vi "SendCmd.vi"(0 "Axis In":T2, 1 "Data Length Constant (0)":u8, 5 "Command":T5 items=["Home Position"=201, "Preset Position"=13, "Soft Overtravel Enable/Disable"=221, "Drive Status"=115, "Position Command"=128, "Run Status"=117, "Fault Status"=116, "Position Error"=129, "Auto-Start Homing"=196, "Start Homing"=205, "Homing Type"=197, "Monitor Index Count"=173, "Motor Position"=126, "Velocity Motor"=133, "Power-Up Status"=1, "Drive Name"=6, "Position Window Size"=22, "Position Window Time"=23, "Zero Speed Limit"=34, "Speed Window Size"=35, "Up to Speed Limit"=37, "Forward Current Limit"=47, "Reverse Current Limit"=48, "Override Mode"=67, "Operation Mode"=90, "Host Control Mode"=97, "Reset Drive"=106, "Drive Enable"=107, "Setpoint Current"=108, "Setpoint Velocity"=109, "Setpoint Acceleration"=110, "Reset Faults"=111, "Position Comparator"=349, "Postition Comparator Polarity"=350, "Position Rollover Enable"=404, "Baud Rate"=80, "Frame Format"=81, "Drive Address"=82, "Broadcast Address"=83, "Auto-start Indexing"=88, "Start Index"=112, "Host Index"=184, "Index Type"=174, "Index Dist/Pos"=175, "Index Reg Dist"=176, "Index Velocity"=177, "Index Acceleration"=178, "Index Deceleration"=179, "Index Dwell"=180, "Index Count"=181, "Index Termination"=182, "Index Pointer"=183, "Index Abort Deceleration"=185, "Positive Soft Pos Limit"=216, "Define Home"=113, "Negative Soft Pos Limit"=217], 7 "Function":T4 items=["Read Working Value", "Write Working Value", "Read Non-Volatile Value", "Write Non-Volatile and Woring Value", "Copy Non-Volatile Value to Working Value", "Copy Working Value to Non-Volatile Value", "Read Default Value", "Copy Default Value to Non-Volatile and Working Values", "Read Min Value", "Read Max Value", "Read Array Index Min", "Read Array Index Max"], 9 "Data (0)":i32, 11 "error in (no error)":errorcluster, 12 "Index (0)":T3) -> (4 "Axis Out":T2, 6 "Data":i32, 10 "Error Message":T1 items=["Invalid Data"=1, "Command Not Enabled"=2, "EEPROM Write Error"=3, "Data Below Min"=4, "Data Above Max"=5, "Command Disabled when Drive Enabled"=6, "Invalid Array Index"=7, "Invalid Function Code"=8, "Invalide Parameter Number"=9], 15 "error out":errorcluster)   [LabVIEW 2009]
uses:
  typedefs/Ultra3000/Cmds.ctl
  typedefs/Ultra3000/Func.ctl
  typedefs/AxisSelect_Enum.ctl
  typedefs/Ultra3000/Index_Numeric.ctl
  typedefs/Ultra3000/Error_Ring.ctl
  globals/AxisSpace.vi
  globals/VISAResourceName.vi
panel:
  out "return count":u32
  out "substring":string
  out "Parameter Field":u32
  out "Received String":string
  out "Input String":string
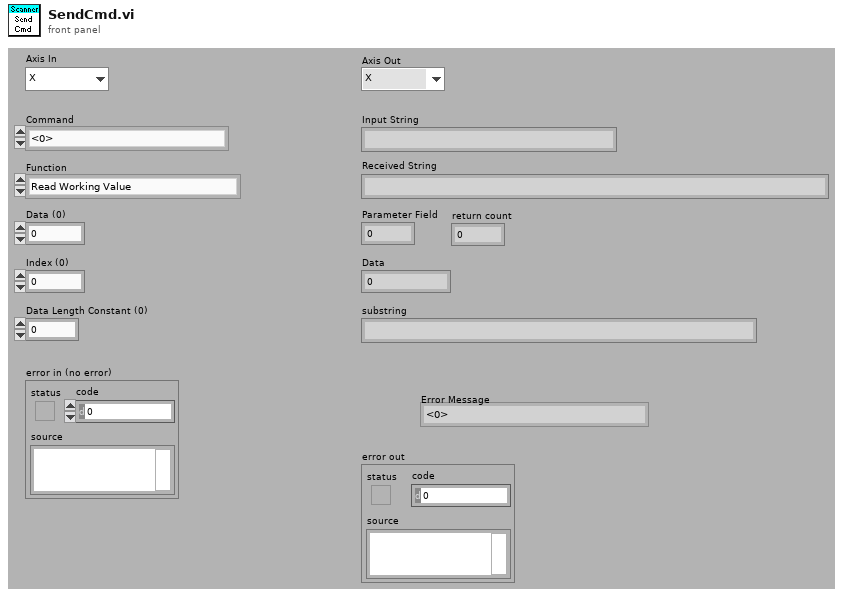
[diagram p1: front panel]
types:
  T1 = typedef "Error_Ring.ctl" = u16
  T2 = typedef "AxisSelect_Enum.ctl" = enum16{"X", "Y", "Z", "Axis Space"}
  T3 = typedef "Index_Numeric.ctl" = u8
  T4 = typedef "Func.ctl" = u16
  T5 = typedef "Cmds.ctl" = u16
  T6 = typedef "AxisSpaceCfg.ctl" = T7[]
  T7 = typedef "AxisCfg.ctl" = cluster{"Addr":u8, "Conv Factor":dbl, "Forward Limit":dbl, "Reverse Limit":dbl, "Enable Limits":bool}
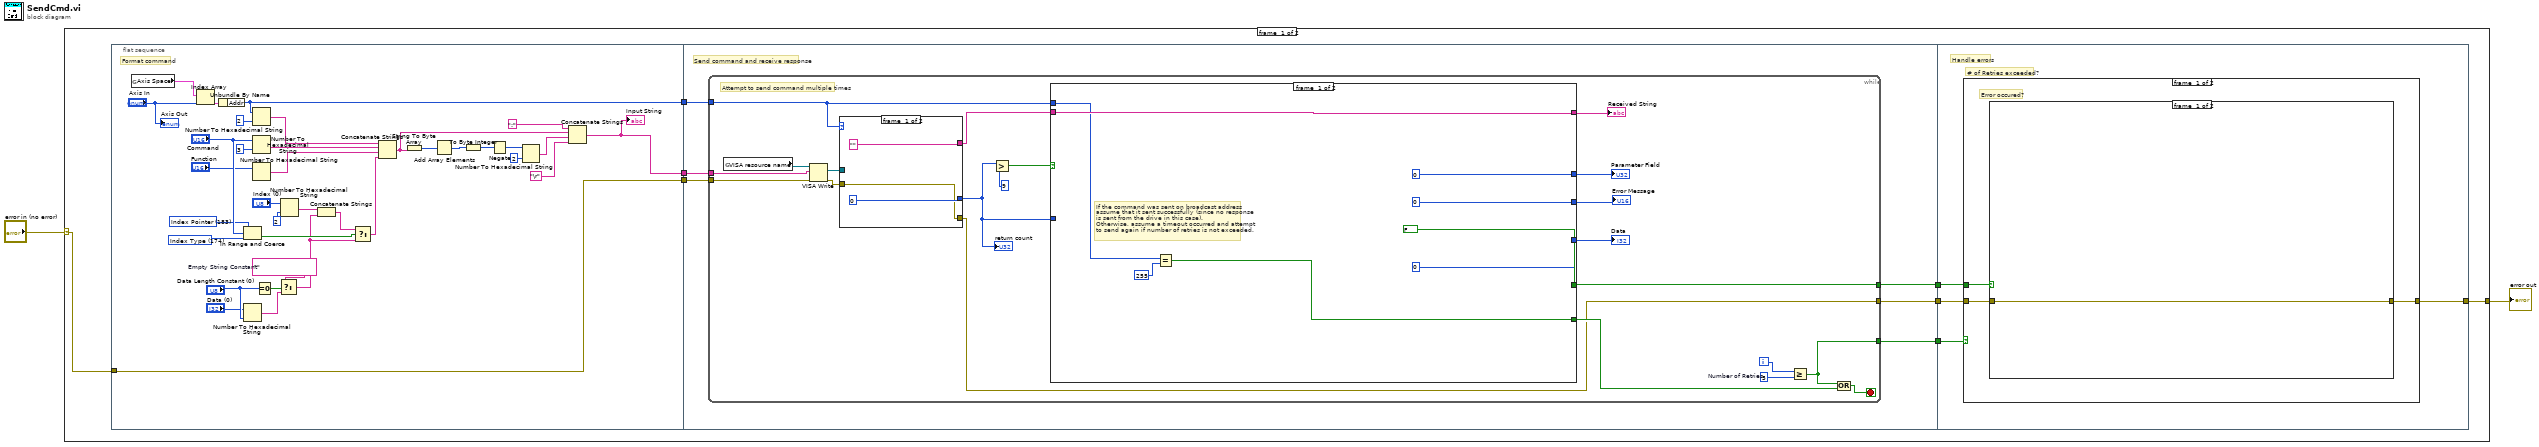
[diagram p0: block diagram]
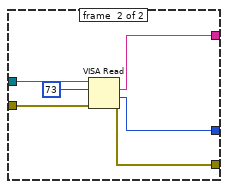
[diagram p2: hidden frame]
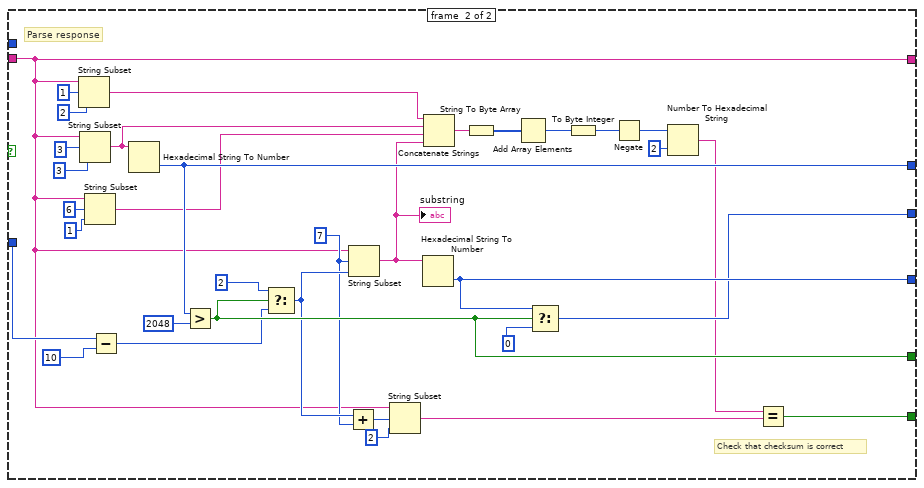
[diagram p3: hidden frame]
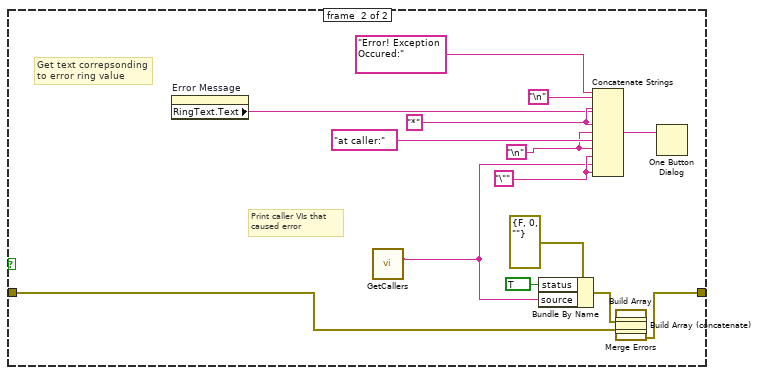
[diagram p4: hidden frame]
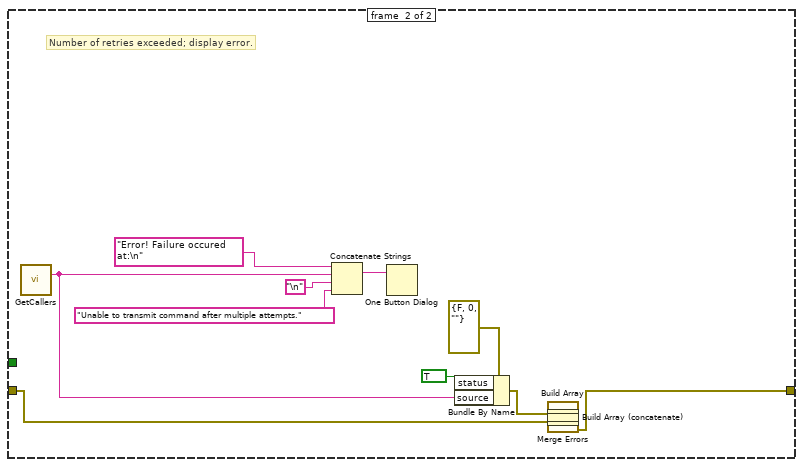
[diagram p5: hidden frame]
diagram:
  n1 = case shown="No Error" "error in (no error)" {
    selector: "error in (no error)" -> [w4 w161]
    tunnel: [w5 w161] -> w2
    frame #0 {
      n2 = flat-sequence {
        tunnel: [w16] -> w9
        tunnel: [w12] -> w10
        tunnel: w4 -> [w11]
        tunnel: [w11] -> w3
        tunnel: w10 -> [w51]
        tunnel: w9 -> [w52]
        tunnel: [w50] -> w8
        tunnel: [w49] -> w7
        tunnel: [w48] -> w6
        tunnel: w3 -> [w47]
        tunnel: w8 -> [w128]
        tunnel: w7 -> [w127]
        tunnel: [w126] -> w5
        tunnel: w6 -> [w125]
        frame #0 {
          w44 = T5 174 items=["Power-Up Status"=1, "Drive Name"=6, "Position Window Size"=22, "Position Window Time"=23, "Zero SPeed Limit"=34, "Speed Window Size"=35, "Up to Speed Limit"=37, "Forward Current Limit"=47, "Reverse Current Limit"=48, "Override Mode"=67, "Operation Mode"=90, "Host Control Mode"=97, "Reset Drive"=106, "Drive Enable"=107, "Setpoint Current"=108, "Setpoint Velocity"=109, "Setpoint Acceleration"=110, "Reset Faults"=111, "Position Comparator"=349, "Postition Comparator Polarity"=350, "Position Rollover Enable"=404, "Baud Rate"=80, "Frame Format"=81, "Drive Address"=82, "Broadcast Address"=83, "Auto-start Indexing"=88, "Start Index"=112, "Host Index"=184, "Index Type"=174, "Index Dist/Pos"=175, "Index Reg Dist"=176, "Index Velocity"=177, "Index Acceleration"=178, "Index Deceleration"=179, "Index Dwell"=180, "Index Count"=181, "Index Termination"=182, "Index Pointer"=183, "Index Abort Deceleration"=185, "Positive Soft Pos Limit"=216, "Negative Soft Pos Limit"=217] ("upper limit")
          w43 = T5 183 items=["Power-Up Status"=1, "Drive Name"=6, "Position Window Size"=22, "Position Window Time"=23, "Zero SPeed Limit"=34, "Speed Window Size"=35, "Up to Speed Limit"=37, "Forward Current Limit"=47, "Reverse Current Limit"=48, "Override Mode"=67, "Operation Mode"=90, "Host Control Mode"=97, "Reset Drive"=106, "Drive Enable"=107, "Setpoint Current"=108, "Setpoint Velocity"=109, "Setpoint Acceleration"=110, "Reset Faults"=111, "Position Comparator"=349, "Postition Comparator Polarity"=350, "Position Rollover Enable"=404, "Baud Rate"=80, "Frame Format"=81, "Drive Address"=82, "Broadcast Address"=83, "Auto-start Indexing"=88, "Start Index"=112, "Host Index"=184, "Index Type"=174, "Index Dist/Pos"=175, "Index Reg Dist"=176, "Index Velocity"=177, "Index Acceleration"=178, "Index Deceleration"=179, "Index Dwell"=180, "Index Count"=181, "Index Termination"=182, "Index Pointer"=183, "Index Abort Deceleration"=185, "Positive Soft Pos Limit"=216, "Negative Soft Pos Limit"=217] ("upper limit")
          w33 = ""  # Empty String Constant
          # "Format command"
          n3 = global read "AxisSpace.vi" "Axis Space"() -> (w15:T6)
          n4 = Index Array(array=w15, index="Axis In") -> (element=w14:T7)
          n5 = Unbundle By Name(w14) -> ("Addr"=w12:u8)
          n6 = In Range and Coerce(upper limit=w43, x="Command", lower limit=w44) -> (In Range?=w42:bool)  [unwired: 1 out]
          n7 = Number To Hexadecimal String(1:"Data Length Constant (0)", 2:"Data (0)") -> (0:w34:string)
          n8 = Number To Hexadecimal String(1:i16 2 ("width (-)"), 2:w12) -> (0:w17:string)
          n9 = Number To Hexadecimal String(1:i16 3 ("width (-)"), 2:"Command") -> (0:w18:string)
          n10 = Number To Hexadecimal String(2:"Function") -> (0:w19:string)  [unwired: 1 in]
          n11 = Equal To 0?(x="Data Length Constant (0)") -> (x = 0?=w32:bool)
          n12 = Select(t=w33, s=w32, f=w34) -> (s? t:f=w40:string)
          n13 = Number To Hexadecimal String(1:i16 2 ("width (-)"), 2:"Index (0)") -> (0:w41:string)
          n14 = Concatenate Strings(w41, w40) -> (w39:string)
          n15 = Select(t=w39, s=w42, f=w40) -> (s? t:f=w37:string)
          n16 = Concatenate Strings(w17, w18, w19, w37) -> (w25:string)
          n17 = String To Byte Array(string=w25) -> (unsigned byte array=w24:u8[])
          n18 = Add Array Elements(numeric array=w24) -> (sum=w27:u8)
          n19 = To Byte Integer(number=w27) -> (8bit integer=w29:i8)
          n20 = Negate(x=w29) -> (-x=w28:i8)
          n21 = Number To Hexadecimal String(1:i16 2 ("width (-)"), 2:w28) -> (0:w30:string)
          n22 = Concatenate Strings(":", w25, w30, "\r") -> (w16:string)
          "Input String" <- w16
          "Axis Out" <- "Axis In"
        }
        frame #1 {
          # "Send command and receive response"
          n23 = while {
            tunnel: [w65] -> w50
            tunnel: w52 -> [w64]
            tunnel: w51 -> [w58]
            tunnel: [w56] -> w49
            tunnel: [w54] -> w48
            tunnel: w47 -> [w53]
            i -> [w59]
            stop <- w60 stop-if-true
            w61 = 5  # Number of Retries
            # "Attempt to send command multiple times"
            n24 = global read "VISAResourceName.vi" "VISA resource name"() -> (w62:refnum<visa-resource-name>)
            n25 = VISA Write(VISA resource name=w62, write buffer=w64, error in (no error)=w53) -> (VISA resource name out=w63:refnum<visa-resource-name>, error out=w55:errorcluster)  [unwired: 1 out]
            n26 = case shown="255" w58 {
              tunnel: w63 -> [_ w81]
              tunnel: ["" ("read buffer") w80] -> w67
              tunnel: [u32 0 ("return count") w79] -> w68
              tunnel: w55 -> [w74 w78]
              tunnel: [w74 w77] -> w54
              frame #0 {
              }
              frame #1 {
                n27 = VISA Read(VISA resource name=w81, byte count=u32 73, error in (no error)=w78) -> (read buffer=w80:string, return count=w79:u32, error out=w77:errorcluster)  [unwired: 1 out]
              }
            }
            "return count" <- w68
            n28 = Greater?(x=w68, y=u32 9) -> (0:w69:bool)
            n29 = case shown="True" w69 {
              tunnel: w67 -> [w86 w98]
              tunnel: [u32 0 w119] -> w70
              tunnel: [u32 0 ("f") w118] -> w66
              tunnel: [u32 0 w117] -> w71
              tunnel: [FALSE w116] -> w65
              tunnel: [w86 w98] -> w72
              tunnel: w68 -> [_ w114]
              tunnel: [w83 w92] -> w57
              tunnel: w58 -> [w85 _]
              frame #0 {
                # "If the command was sent on broadcast address\nassume that it sent successfully (since no response\nis sent from the drive in this case).\nOtherwise, assume a timeout occurred and attempt\nto send again if number of retries is not exceeded."
                n30 = Equal?(x=w85, y=u8 255) -> (x = y?=w83:bool)
              }
              frame #1 {
                w101 = 7 ("offset (0)")
                # "Check that checksum is correct"
                # "Parse response"
                n31 = String Subset(string=w98, offset (0)=1, length (rest)=2 ("length (rest)")) -> (substring=w91:string)
                n32 = String Subset(string=w98, offset (0)=3, length (rest)=3 ("length (rest)")) -> (substring=w97:string)
                n33 = String Subset(string=w98, offset (0)=6, length (rest)=1 ("length (rest)")) -> (substring=w96:string)
                n34 = Subtract(x=w114, y=u32 10) -> (x-y=w115:u32)
                n35 = Hexadecimal String To Number(string=w97) -> (number=w117:u32)  [unwired: 2 in, 1 out]
                n36 = Greater?(x=w117, y=u32 2048) -> (0:w116:bool)
                n37 = Select(t=u8 2, s=w116, f=w115) -> (s? t:f=w102:u32)
                n38 = Add(x=w102, y=w101) -> (x+y=w112:u32)
                n39 = String Subset(string=w98, offset (0)=w101, length (rest)=w102) -> (substring=w95:string)
                "substring" <- w95
                n40 = String Subset(string=w98, offset (0)=w112, length (rest)=2 ("length (rest)")) -> (substring=w94:string)
                n41 = Hexadecimal String To Number(string=w95) -> (number=w119:u32)  [unwired: 2 in, 1 out]
                n42 = Concatenate Strings(w91, w97, w96, w95) -> (w103:string)
                n43 = String To Byte Array(string=w103) -> (unsigned byte array=w105:u8[])
                n44 = Add Array Elements(numeric array=w105) -> (sum=w106:u8)
                n45 = Select(t=w119, s=w116, f=u32 0) -> (s? t:f=w118:u32)
                n46 = To Byte Integer(number=w106) -> (8bit integer=w108:i8)
                n47 = Negate(x=w108) -> (-x=w107:i8)
                n48 = Number To Hexadecimal String(1:i16 2 ("width (-)"), 2:w107) -> (0:w93:string)
                n49 = Equal?(x=w93, y=w94) -> (x = y?=w92:bool)
              }
            }
            "Data" <- w70
            "Parameter Field" <- w71
            "Received String" <- w72
            "Error Message" <- w66
            n50 = Greater Or Equal?(x=w59, y=w61) -> (x >= y?=w56:bool)
            n51 = Compound Arithmetic op=OR(w56, w57) -> (w60:bool)
          }
        }
        frame #2 {
          # "# of Retries exceeded?"
          # "Handle errors"
          n52 = case shown="False" w127 {
            tunnel: w128 -> [w131 _]
            tunnel: [w130 w151] -> w126
            tunnel: w125 -> [w129 w152]
            frame #0 {
              # "Error occured?"
              n53 = case shown="True" w131 {
                tunnel: [w132 w136] -> w130
                tunnel: w129 -> [w132 w135]
                frame #0 {
                }
                frame #1 {
                  w142 = "\n"
                  w143 = "\"" ("string")
                  w147 = "*" ("string")
                  # "Print caller VIs that\ncaused error"
                  # "Get text correpsonding \nto error ring value"
                  n54 = property on="Error Message" class="Ring (strict)"() -> ("RingText.Text"=w141:string)  [unwired: 2 in, 2 out]
                  n55 = call "GetCallers.vi"() -> ("Caller String"=w138:string)  [unwired: 15 in]
                  n56 = Bundle By Name(cluster=errorcluster {"status"=FALSE, "code"=0, "source"=""} ("error out"), "status"=TRUE, "source"=w138) -> (w137:errorcluster)
                  n57 = Concatenate Strings("Error! Exception Occured:", "\n", w147, w141, w147, w142, "at caller:" ("string"), w142, w143, w138, w143) -> (w148:string)
                  n58 = Build Array(w137, w135) -> (w134:errorcluster[])
                  n59 = Build Array (concatenate)(w134) -> (w133:errorcluster[])
                  n60 = call <vilib>:"Merge Errors.vi"("error array in"=w133) -> ("error out"=w136:errorcluster)  [unwired: 6 in]
                  n61 = One Button Dialog(message=w148) -> ()  [unwired: 1 in, 1 out]
                }
              }
            }
            frame #1 {
              # "Number of retries exceeded; display error."
              n62 = call "GetCallers.vi"() -> ("Caller String"=w154:string)  [unwired: 15 in]
              n63 = Concatenate Strings("Error! Failure occured at:\n" ("message"), w154, "\n", "Unable to transmit command after multiple attempts." ("string")) -> (w160:string)
              n64 = One Button Dialog(message=w160) -> ()  [unwired: 1 in, 1 out]
              n65 = Bundle By Name(cluster=errorcluster {"status"=FALSE, "code"=0, "source"=""} ("error out"), "status"=TRUE, "source"=w154) -> (w153:errorcluster)
              n66 = Build Array(w153, w152) -> (w150:errorcluster[])
              n67 = Build Array (concatenate)(w150) -> (w149:errorcluster[])
              n68 = call <vilib>:"Merge Errors.vi"("error array in"=w149) -> ("error out"=w151:errorcluster)  [unwired: 6 in]
            }
          }
        }
      }
    }
    frame #1 {
    }
  }
  "error out" <- w2
